vi "DLL Connect and Read Config.vi"(8 "error in (no error)":errorcluster, 11 "Phasor Data Concentrator in":refnum<class "Phasor Data Concentrator.lvclass">) -> (0 "error out":errorcluster, 3 "Phasor Data Concentrator out":refnum<class "Phasor Data Concentrator.lvclass">)   [LabVIEW 2013, in "PMU Recorder Light.lvlib" / "Phasor Data Concentrator.lvclass"]
doc: "Calls the DLL class to connect to the PDC."
uses:
  Phasor Data Concentrator.lvclass
  PMU Recorder Light.lvlib
  Setting Choice.ctl
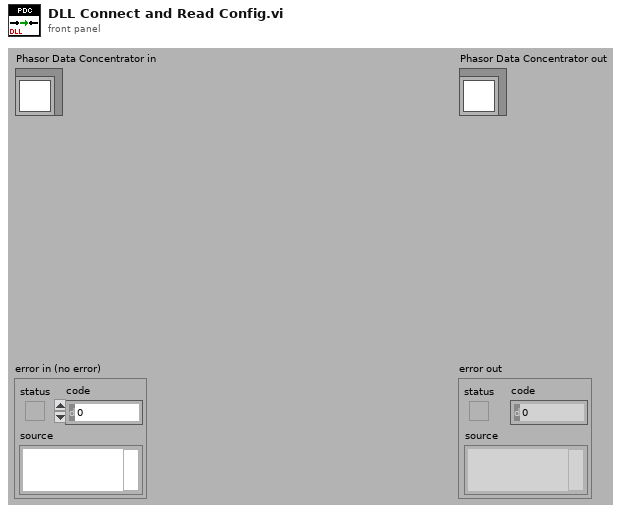
[diagram p1: front panel]
types:
  T1 = typedef "PMU Recorder Light.lvlib/Setting Choice.ctl" = enum16{"Analog Data Points Allowed Equals", "Complex Data Points Allowed Equals", "Seconds Before Reset After Wait for Config Fails", "Number of Live Buffer in Access Buffer ", "Number of Connection Attempts", "Live Data Buffer Size", "dt Tolerance", "Data Rate History", "ALL"}
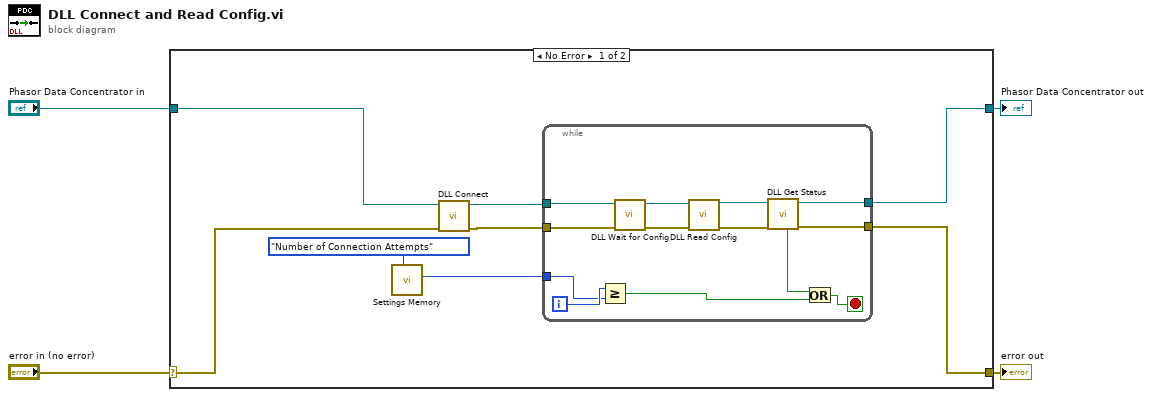
[diagram p0: block diagram]
diagram:
  n1 = case shown="No Error" "error in (no error)" {
    selector: "error in (no error)" -> [w7 w27]
    tunnel: [w12 w27] -> w3
    tunnel: [w11 w26] -> w1
    tunnel: "Phasor Data Concentrator in" -> [w8 w26]
    frame No Error {
      n2 = call "Settings Memory.vi"("Setting Choice"=Setting_Choice."Number of Connection Attempts") -> ("Output Int32"=w5:i32)  [unwired: 8 in, 2 out]
      n3 = call "DLL Connect.vi"("error in (no error)"=w7, "Phasor Data Concentrator in"=w8) -> ("error out"=w9:errorcluster, "Phasor Data Concentrator out"=w10:refnum<class "Phasor Data Concentrator.lvclass">)  [unwired: 8 in]
      n4 = while {
        tunnel: w10 -> [w14]
        tunnel: w9 -> [w13]
        tunnel: [w21] -> w12
        tunnel: [w20] -> w11
        tunnel: w5 -> [w18]
        i -> [w19]
        stop <- w15 stop-if-true
        n5 = Greater Or Equal?(x=w19, y=w18) -> (x >= y?=w16:bool)
        n6 = call "DLL Wait for Config.vi"("error in (no error)"=w13, "Phasor Data Concentrator in"=w14) -> ("error out"=w24:errorcluster, "Phasor Data Concentrator out"=w25:refnum<class "Phasor Data Concentrator.lvclass">)  [unwired: 8 in]
        n7 = call "DLL Read Config.vi"("error in (no error)"=w24, "Phasor Data Concentrator in"=w25) -> ("error out"=w22:errorcluster, "Phasor Data Concentrator out"=w23:refnum<class "Phasor Data Concentrator.lvclass">)  [unwired: 8 in]
        n8 = call "DLL Get Status.vi"("error in (no error)"=w22, "Phasor Data Concentrator in"=w23) -> ("error out"=w21:errorcluster, "Phasor Data Concentrator out"=w20:refnum<class "Phasor Data Concentrator.lvclass">, "Configuration Read OK"=w17:bool)  [unwired: 3 in, 4 out]
        n9 = Or(x=w17, y=w16) -> (x .or. y?=w15:bool)
      }
    }
    frame Error {
    }
  }
  "error out" <- w3
  "Phasor Data Concentrator out" <- w1
